vi "Flex UI.vi"() -> ()   [LabVIEW 2016]
uses:
  Source/FlexUIActorMaker.lvclass
panel:
  in  "Flex UI Class Name":string caption="String"
  in  "Destination":path caption="Path"
  in  "OK Button":bool
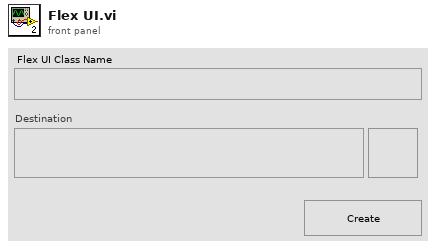
[diagram p1: front panel]
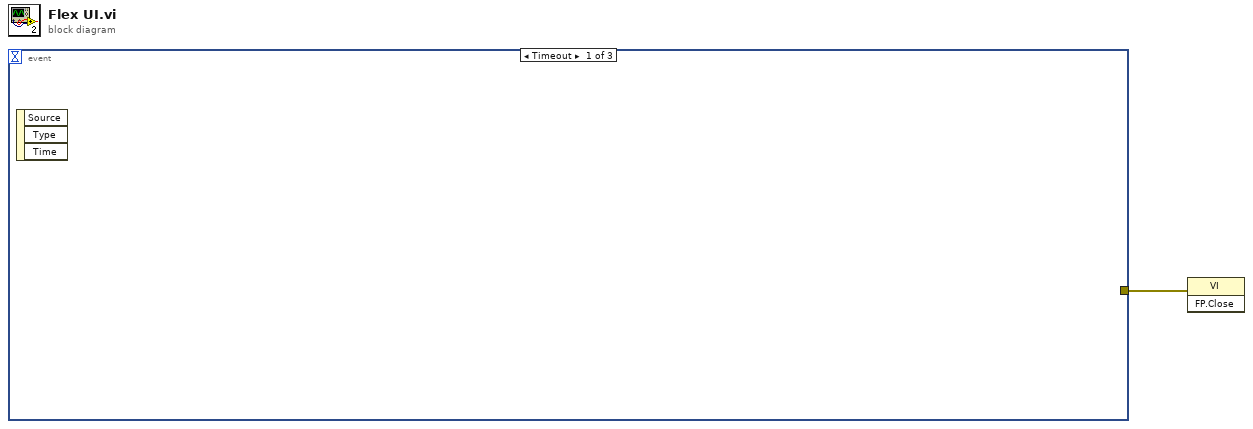
[diagram p0: block diagram]
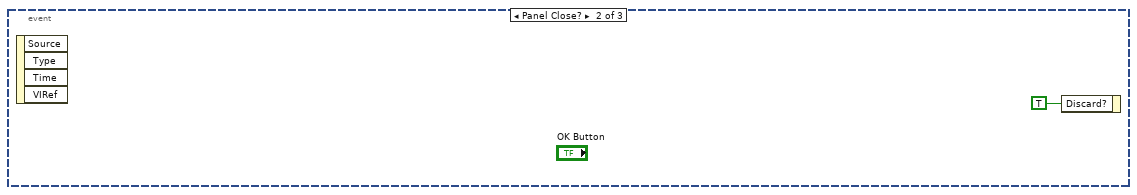
[diagram p2: hidden frame]
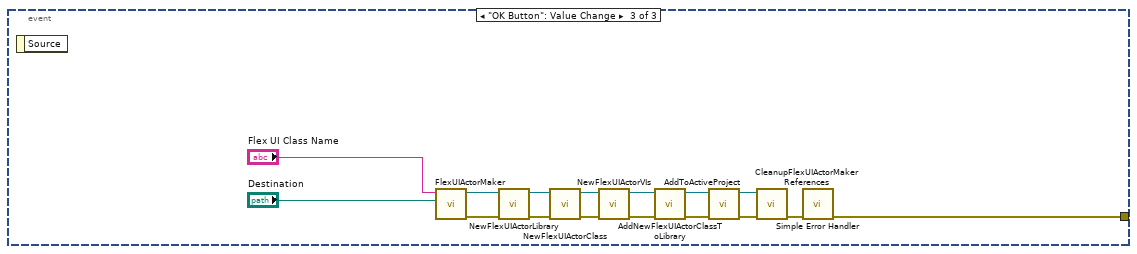
[diagram p3: hidden frame]
diagram:
  n1 = event shown="[0] Timeout" {
    selector: _ -> [_ _ _]
    dyn-events: _ -> [_ _ _]
    timeout: _ -> [_ _ _]
    tunnel: [_ _ w3] -> w1
    event Timeout {
      n2 = event-data() -> ()  [unwired: 1 in, 3 out]
    }
    event Panel Close? {
      n3 = event-data() -> ()  [unwired: 1 in, 4 out]
      n4 = event-data("Discard?"=TRUE) -> ()  [unwired: 1 in, 1 out]
    }
    event "OK Button": Value Change {
      n5 = event-data() -> ()  [unwired: 1 in, 1 out]
      n6 = call "FlexUIActorMaker.vi"("UIClassDestination"="Destination", "UIClassName"="Flex UI Class Name") -> ("error out"=w12:errorcluster, "FlexUIActorMaker.lvlib:FlexUIActorMaker.lvclass"=w13:refnum<class "FlexUIActorMaker.lvclass">)  [unwired: 8 in]
      n7 = call-dynamic "NewFlexUIActorLibrary.vi"("error in (no error)"=w12, "FlexUIActorMaker in"=w13) -> ("error out"=w11:errorcluster, "FlexUIActorMaker out"=w10:refnum<class "FlexUIActorMaker.lvclass">)  [unwired: 8 in]
      n8 = call-dynamic "NewFlexUIActorClass.vi"("error in (no error)"=w11, "FlexUIActorMaker in"=w10) -> ("error out"=w18:errorcluster, "FlexUIActorMaker out"=w17:refnum<class "FlexUIActorMaker.lvclass">)  [unwired: 8 in]
      n9 = call-dynamic "NewFlexUIActorVIs.vi"("error in (no error)"=w18, "FlexUIActorMaker in"=w17) -> ("error out"=w8:errorcluster, "FlexUIActorMaker out"=w9:refnum<class "FlexUIActorMaker.lvclass">)  [unwired: 8 in]
      n10 = call-dynamic "AddNewFlexUIActorClassToLibrary.vi"("error in (no error)"=w8, "FlexUIActorMaker in"=w9) -> ("error out"=w7:errorcluster, "FlexUIActorMaker out"=w6:refnum<class "FlexUIActorMaker.lvclass">)  [unwired: 8 in]
      n11 = call-dynamic "AddToActiveProject.vi"("error in (no error)"=w7, "FlexUIActorMaker in"=w6) -> ("error out"=w16:errorcluster, "FlexUIActorMaker out"=w15:refnum<class "FlexUIActorMaker.lvclass">)  [unwired: 8 in]
      n12 = call-dynamic "CleanupFlexUIActorMakerReferences.vi"("error in (no error)"=w16, "FlexUIActorMaker in"=w15) -> ("error out"=w14:errorcluster)  [unwired: 8 in, 1 out]
      n13 = call <vilib>:"Simple Error Handler.vi"("error in (no error)"=w14) -> ("error out"=w3:errorcluster)  [unwired: 4 in, 4 out]
    }
  }
  n14 = invoke class="VI" method="FP.Close"(error in=w1) -> ()  [unwired: 2 in, 3 out]
